vi "Coerce Repetition Rate (scalar).vi"(9 "Npts":i32, 10 "Sampling rate (Hz)":dbl, 11 "Rep Rate (Hz)":dbl) -> (3 "Coerced Rep Rate (Hz)":dbl)   [LabVIEW 2020]
panel:
  out "coerced pts/period":i32
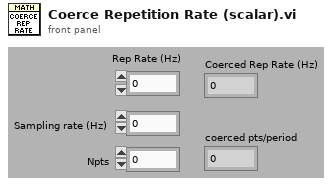
[diagram p1: front panel]
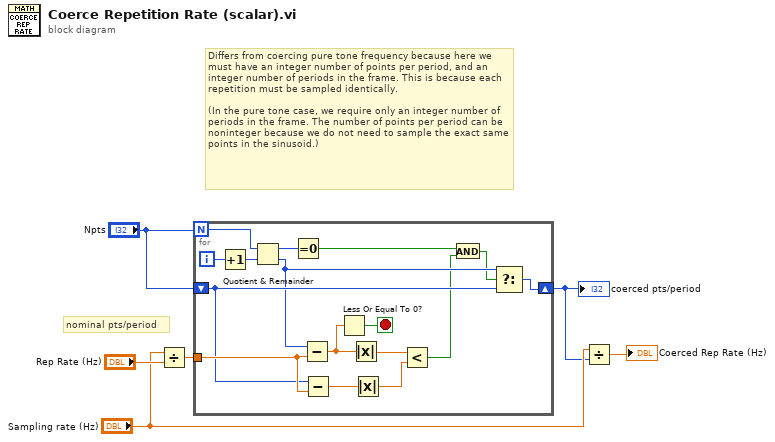
[diagram p0: block diagram]
diagram:
  # "nominal pts/period"
  # "Differs from coercing pure tone frequency because here we must have an integer number of points per period, and an integer number of periods in the frame. This is because each repetition must be sampled identically. \n\n(In the pure tone case, we require only an integer number of periods in the frame. The number of points per period can be noninteger because we do not need to sample the exact same points in the sinusoid.)"
  n1 = Divide(x="Sampling rate (Hz)", y="Rep Rate (Hz)") -> (x/y=w4:dbl)
  n2 = for {
    N: "Npts" -> [w22]
    tunnel: w4 -> [w17]
    shift-right: [w13] -> w2
    shift-left: "Npts" -> [w12]
    i -> [w7]
    stop <- w19 stop-if-true
    n3 = Increment(x=w7) -> (x+1=w20:i32)
    n4 = Quotient & Remainder(x=w22, y=w20) -> (x-y*floor(x/y)=w21:i32, floor(x/y)=w11:i32)
    n5 = Equal To 0?(x=w21) -> (x = 0?=w8:bool)
    n6 = Subtract(x=w11, y=w17) -> (x-y=w18:dbl)
    n7 = Subtract(x=w12, y=w17) -> (x-y=w16:dbl)
    n8 = Less Or Equal To 0?(x=w18) -> (x <= 0?=w19:bool)
    n9 = Absolute Value(x=w18) -> (abs(x)=w15:dbl)
    n10 = Absolute Value(x=w16) -> (abs(x)=w14:dbl)
    n11 = Less?(x=w15, y=w14) -> (x < y?=w9:bool)
    n12 = And(x=w8, y=w9) -> (x .and. y?=w10:bool)
    n13 = Select(t=w11, s=w10, f=w12) -> (s? t:f=w13:i32)
  }
  "coerced pts/period" <- w2
  n14 = Divide(x="Sampling rate (Hz)", y=w2) -> (x/y=→"Coerced Rep Rate (Hz)":dbl)
